vi "Save-Load General Setup Parameters.vi"(6 "backup file path":path, 8 "error in":errorcluster, 11 "Function":T1=enum."Load from file") -> (0 "error out":errorcluster)   [LabVIEW 2020]
uses:
  Typedefs/Save-Load enum.ctl
  Typedefs/Which path.ctl
  <vilib>/Utility/config.llb/NI_LVConfig.lvlib
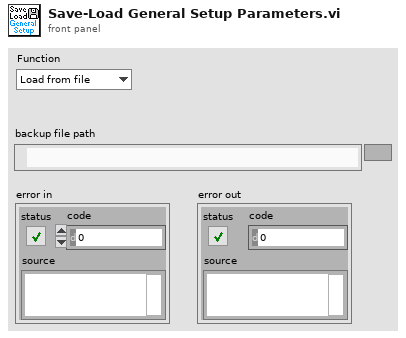
[diagram p1: front panel]
types:
  T1 = typedef "Save-Load enum.ctl" = enum16{"Save to file", "Load from file", "Compare from file", "Save Backup"}
  T2 = typedef "Which path.ctl" = enum16{"Configuration Files", "Calibration Files", "Images", "Setup.ini", "Loaded User profile.ini", "User's-Previous session.ini", "New user profile.ini", "Selected User profile.ini", "User profiles folder", "Power meter scaling.txt", "FOV Cal.ini", "Calibration.ini"}
  T3 = typedef "NI_LVConfig.lvlib/Config Data RefNum.ctl" = refnum<k1>
  T4 = typedef "Ini file interface (DBL).ctl" = cluster{"key":string, "Save?":bool, "Default":dbl}[]
  T5 = typedef "Ini file interface (String).ctl" = cluster{"key":string, "Save?":bool, "Default":string}[]
  T6 = typedef "Ini file interface (Boolean).ctl" = cluster{"key":string, "Save?":bool, "Default":bool}[]
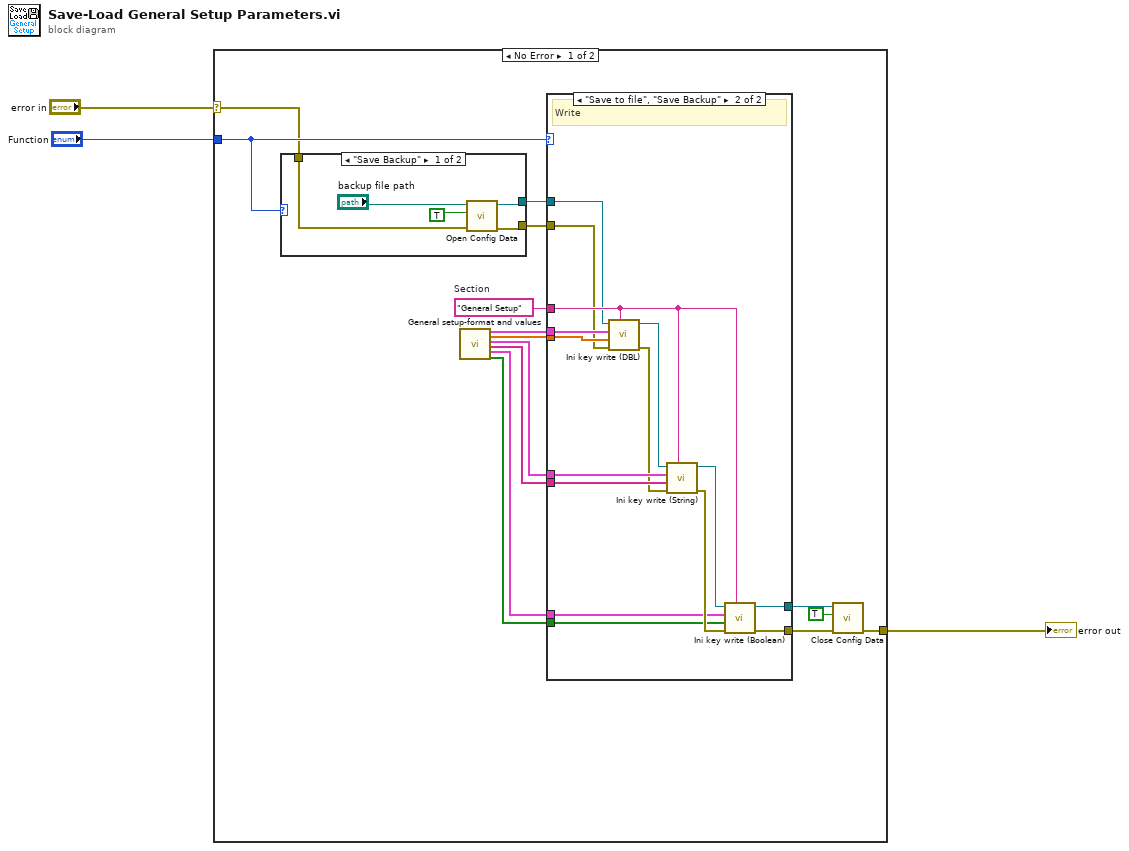
[diagram p0: block diagram]
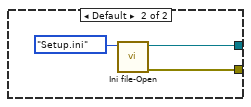
[diagram p2: hidden frame]
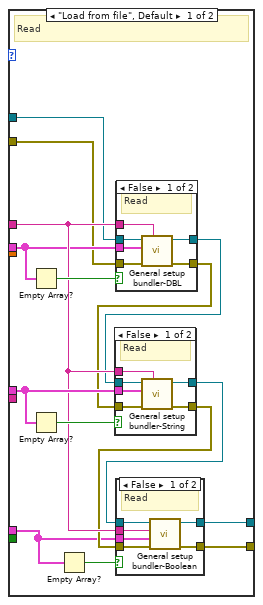
[diagram p3: hidden frame]
diagram:
  n1 = case shown="No Error" "error in" {
    selector: "error in" -> [w4 w81]
    tunnel: [w7 w81] -> w3
    tunnel: "Function" -> [w5 _]
    frame No Error {
      w18 = "General Setup"  # Section
      n2 = case shown="\"Save Backup\"" w5 {
        tunnel: [w19 w26] -> w16
        tunnel: [w20 w25] -> w15
        tunnel: w4 -> [w21 _]
        frame "Save Backup" {
          n3 = call <vilib>:"Open Config Data.vi"("error in (no error)"=w21, "create file if necessary (T)"=TRUE ("create file if necessary"), "configuration file path"="backup file path") -> ("error out"=w20:errorcluster, "refnum"=w19:T3)  [unwired: 6 in, 1 out]
        }
        frame Default {
          n4 = call "Ini file-Open.vi"("Which file?"=Which_path."Setup.ini") -> ("error out"=w25:errorcluster, "User profile ini file ref"=w26:T3)  [unwired: 7 in, 2 out]
        }
      }
      n5 = call "General setup-format and values.vi"() -> ("DBL"=w13:T4, "DBL values"=w12:dbl[], "String"=w11:T5, "String values"=w10:string[], "Boolean"=w9:T6, "Boolean values"=w8:bool[])  [unwired: 14 in]
      n6 = case shown="\"Save to file\", \"Save Backup\"" w5 {
        tunnel: [w39 w71] -> w6
        tunnel: [w40 w70] -> w14
        tunnel: w15 -> [w30 w66]
        tunnel: w16 -> [w31 w67]
        tunnel: w18 -> [w35 w73]
        tunnel: w12 -> [_ w75]
        tunnel: w8 -> [_ w69]
        tunnel: w10 -> [_ w79]
        tunnel: w11 -> [w36 w80]
        tunnel: w13 -> [w32 w76]
        tunnel: w9 -> [w29 w68]
        frame "Load from file", Default {
          # "Read"
          n7 = Empty Array?(array=w32) -> (empty?=w41:bool)
          n8 = Empty Array?(array=w36) -> (empty?=w37:bool)
          n9 = Empty Array?(array=w29) -> (empty?=w38:bool)
          n10 = case shown="False" w41 {
            tunnel: [w62 w65] -> w27
            tunnel: [w63 w64] -> w28
            tunnel: w32 -> [w58 _]
            tunnel: w31 -> [w61 w65]
            tunnel: w30 -> [w60 w64]
            tunnel: w35 -> [w59 _]
            frame False {
              # "Read"
              n11 = call "General setup bundler-DBL.vi"("Section"=w59, "error in (no error)"=w60, "DBL"=w58, "Setup.ini ref"=w61) -> ("error out"=w63:errorcluster, "Setup.ini ref"=w62:T3)  [unwired: 6 in]
            }
            frame True {
              # "No parametersof such type"
            }
          }
          n12 = case shown="False" w37 {
            tunnel: [w46 w49] -> w34
            tunnel: [w45 w48] -> w33
            tunnel: w36 -> [w43 _]
            tunnel: w27 -> [w47 w49]
            tunnel: w28 -> [w44 w48]
            tunnel: w35 -> [w42 _]
            frame False {
              # "Read"
              n13 = call "General setup bundler-String.vi"("Section"=w42, "error in (no error)"=w44, "String"=w43, "Setup.ini ref"=w47) -> ("error out"=w45:errorcluster, "Setup.ini ref"=w46:T3)  [unwired: 6 in]
            }
            frame True {
              # "No parametersof such type"
            }
          }
          n14 = case shown="False" w38 {
            tunnel: [w54 w57] -> w40
            tunnel: [w50 w56] -> w39
            tunnel: w34 -> [w55 w57]
            tunnel: w33 -> [w51 w56]
            tunnel: w35 -> [w53 _]
            tunnel: w29 -> [w52 _]
            frame False {
              # "Read"
              n15 = call "General setup bundler-Boolean.vi"("error in (no error)"=w51, "Boolean"=w52, "Section"=w53, "Setup.ini ref"=w55) -> ("error out"=w50:errorcluster, "Setup.ini ref"=w54:T3)  [unwired: 6 in]
            }
            frame True {
              # "No parametersof such type"
            }
          }
        }
        frame "Save to file", "Save Backup" {
          # "Write"
          n16 = call "Ini key write (DBL).vi"("Section"=w73, "error in (no error)"=w66, "Values (DBL)"=w75, "Ini file interface"=w76, "Ini file refnum in"=w67) -> ("error out"=w78:errorcluster, "Ini file refnum out"=w77:T3)  [unwired: 5 in]
          n17 = call "Ini key write (String).vi"("Section"=w73, "error in (no error)"=w78, "Values (String)"=w79, "Ini file interface"=w80, "Ini file refnum in"=w77) -> ("error out"=w72:errorcluster, "Ini file refnum out"=w74:T3)  [unwired: 5 in]
          n18 = call "Ini key write (Boolean).vi"("Section"=w73, "error in (no error)"=w72, "Values (Boolean)"=w69, "Ini file interface"=w68, "Ini file refnum in"=w74) -> ("error out"=w71:errorcluster, "Ini file refnum out"=w70:T3)  [unwired: 5 in]
        }
      }
      n19 = call <vilib>:"Close Config Data.vi"("error in (no error)"=w6, "write file if changed (T)"=TRUE ("write configuration file? (F)"), "refnum"=w14) -> ("error out"=w7:errorcluster)  [unwired: 7 in, 1 out]
    }
    frame Error {
    }
  }
  "error out" <- w3
